vi "sc_write_data_time.vi"(6 "Value":dbl, 7 "Spare":dbl, 9 "Name":string, 10 "Spill Number":i32, 11 "stripped path":path) -> (3 "String":string)   [LabVIEW 2018]
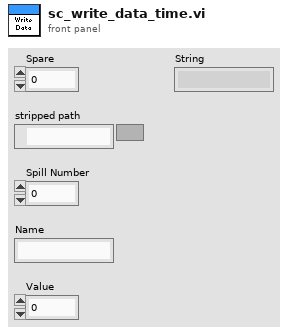
[diagram p1: front panel]
types:
  T1 = enum16{"open", "replace", "create", "open or create", "replace or create", "replace or create with confirmation"}
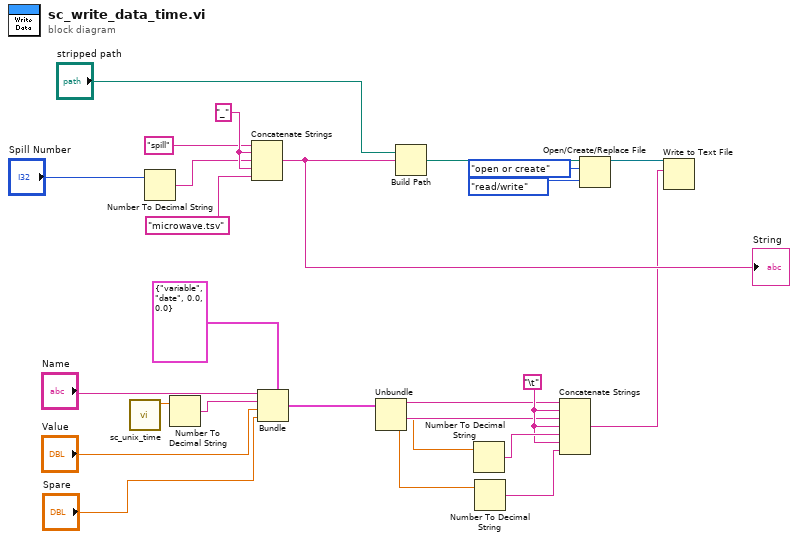
[diagram p0: block diagram]
diagram:
  w19 = "_"
  w10 = "\t"
  n1 = call "sc_unix_time.vi"() -> ("Numeric"=w25:dbl)  [unwired: 10 in, 1 out]
  n2 = Number To Decimal String(number="Spill Number") -> (decimal integer string=w18:string)  [unwired: 1 in]
  n3 = Number To Decimal String(number=w25) -> (decimal integer string=w26:string)  [unwired: 1 in]
  n4 = Concatenate Strings("spill", w19, w18, w19, "microwave.tsv") -> (w21:string)
  "String" <- w21
  n5 = Bundle(cluster=cluster{string, "date string":string, dbl, dbl} {"variable", "date string"="date", 0.0, 0.0}, "Name", "date string"=w26, "Value", "Spare") -> (w5:cluster{string, "date string":string, dbl, dbl})
  n6 = Unbundle(w5) -> (w8:string, "date string"=w9:string, w6:dbl, w7:dbl)
  n7 = Build Path(base path="stripped path", name or relative path=w21) -> (appended path=w22:path)
  n8 = Number To Decimal String(number=w6) -> (decimal integer string=w11:string)  [unwired: 1 in]
  n9 = Number To Decimal String(number=w7) -> (decimal integer string=w12:string)  [unwired: 1 in]
  n10 = Concatenate Strings(w8, w10, w9, w10, w11, w10, w12) -> (w13:string)
  n11 = Open/Create/Replace File(file path (use dialog)=w22, operation (0:open)=T1."open or create", access (0:read/write)=enum16{"read/write", "read-only", "write-only"}."read/write") -> (refnum out=w3:refnum<file>)  [unwired: 3 in, 2 out]
  n12 = Write to Text File(file (use dialog)=w3, text=w13) -> ()  [unwired: 2 in, 3 out]
